vi "Format Address Pads.vi"(4 "WorkTable":refnum<class "WorkTable Class.lvclass">, 6 "Sides":T1[](array[typedef]), 8 "error in":errorcluster, 9 "Slot":i32, 10 "Chuck":i32, 11 "Console Log in":refnum<class "Console Log.lvclass">) -> (0 "error out":errorcluster, 2 "Formatted Address Pads":string[](array[string]), 3 "Console Log out":refnum<class "Console Log.lvclass">)   [LabVIEW 2011, in "Console Log.lvclass"]
uses:
  Console Log.lvclass
  Shared Components/Utils/Type Definitions/3d Line.ctl
  Shared Components/Vec3d Class/Vec3d Class.lvclass
  Shared Components/WorkTable Class/WorkTable Class.lvclass
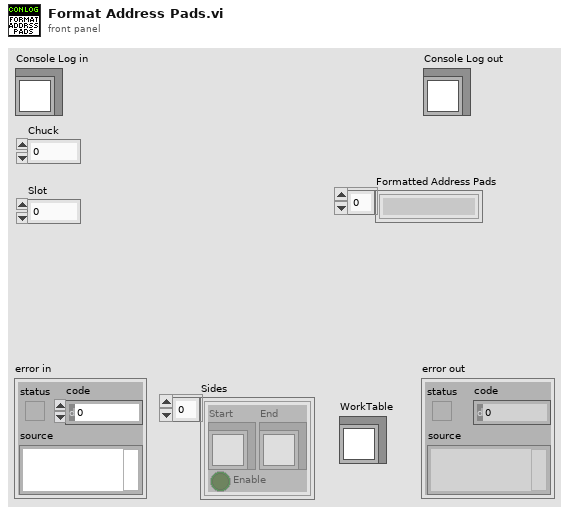
[diagram p1: front panel]
types:
  T1 = typedef "3d Line.ctl" = cluster{"Start":refnum<class "Vec3d Class.lvclass">, "End":refnum<class "Vec3d Class.lvclass">, "Enable":bool}
  T2 = typedef "Worktable_Module Slot.ctl" = cluster{"Slot State":enum16{"Empty", "Bare HDI", "Unglued", "Stamped", "PartOnTop", "Weighted", "Unpotted", "Potted"}, "BBM Type":enum16{"None", "BBM", "GlassSlide"}, "HDI Type":enum16{"None", "HDI", "Polyimide"}, "Vacuum Channel":u8, "Location/Orientation BBM":T3, "Location/Orientation HDI":T3, "S/N":string}
  T3 = typedef "Position_Orientation.ctl" = cluster{"Center":refnum<class "Vec3d Class.lvclass">, "Orientation":refnum<class "Orient3d Class.lvclass">}
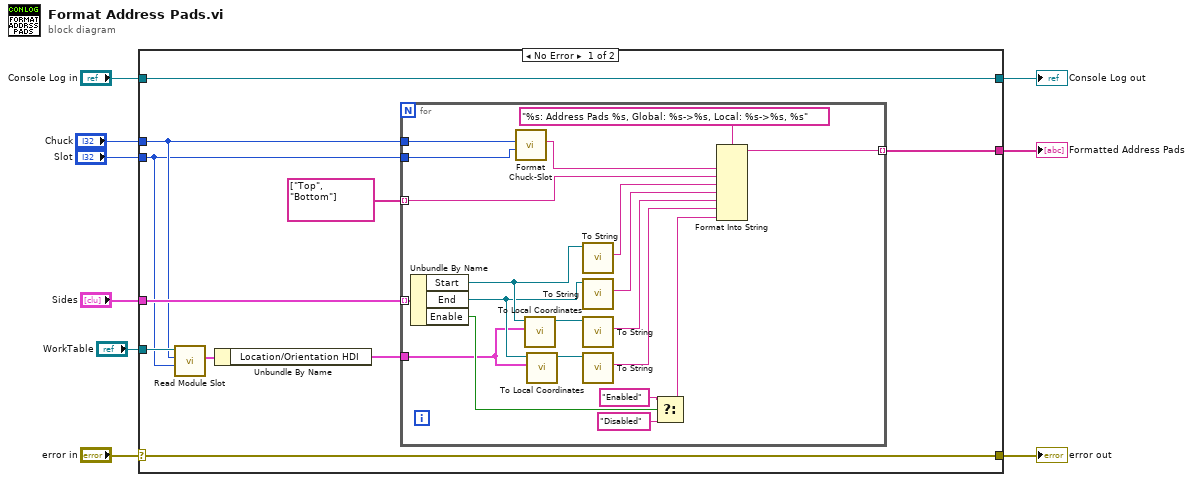
[diagram p0: block diagram]
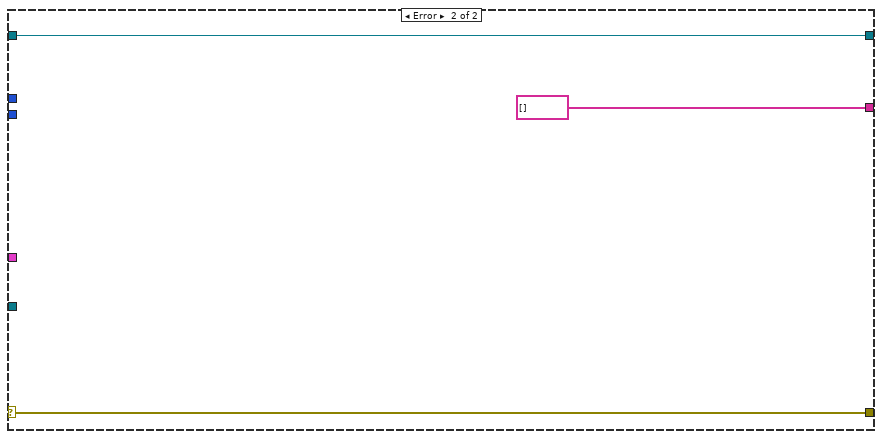
[diagram p2: hidden frame]
diagram:
  n1 = case shown="No Error" "error in" {
    selector: "error in" -> [w18 w42]
    tunnel: [w18 w42] -> w8
    tunnel: [w19 w41] -> w6
    tunnel: "Console Log in" -> [w19 w41]
    tunnel: "Sides" -> [w17 _]
    tunnel: [w16 string[] []] -> w4
    tunnel: "Chuck" -> [w13 _]
    tunnel: "Slot" -> [w12 _]
    tunnel: "WorkTable" -> [w14 _]
    frame No Error {
      n2 = call-dynamic "Read Module Slot.vi"("slot"=w12, "chuck"=w13, "WorkTable in"=w14) -> ("Module Slot"=w11:T2)  [unwired: 6 in, 2 out]
      n3 = Unbundle By Name(w11) -> ("Location/Orientation HDI"=w10:T3)
      n4 = for {
        tunnel: w17 -> [w39] mode=indexing
        tunnel: [w32] -> w16 mode=indexing
        tunnel: string[] ["Top", "Bottom"] -> [w31] mode=indexing
        tunnel: w13 -> [w28]
        tunnel: w12 -> [w27]
        tunnel: w10 -> [w22]
        n5 = Unbundle By Name(w39) -> ("Start"=w24:refnum<class "Vec3d Class.lvclass">, "End"=w23:refnum<class "Vec3d Class.lvclass">, "Enable"=w38:bool)
        n6 = call "Format Chuck-Slot.vi"("Slot"=w27, "Chuck"=w28) -> ("Formatted Chuck/Slot"=w30:string)  [unwired: 7 in, 2 out]
        n7 = call "To Local Coordinates.vi"("Center/Orientation"=w22, "Global Coordinates"=w24) -> ("Local Coordinates"=w26:refnum<class "Vec3d Class.lvclass">)  [unwired: 8 in, 1 out]
        n8 = call "To Local Coordinates.vi"("Center/Orientation"=w22, "Global Coordinates"=w23) -> ("Local Coordinates"=w25:refnum<class "Vec3d Class.lvclass">)  [unwired: 8 in, 1 out]
        n9 = call "To String.vi"("Vec3d in"=w24) -> ("Vec3d String"=w34:string)  [unwired: 8 in, 2 out]
        n10 = call "To String.vi"("Vec3d in"=w23) -> ("Vec3d String"=w33:string)  [unwired: 8 in, 2 out]
        n11 = call "To String.vi"("Vec3d in"=w26) -> ("Vec3d String"=w21:string)  [unwired: 8 in, 2 out]
        n12 = call "To String.vi"("Vec3d in"=w25) -> ("Vec3d String"=w20:string)  [unwired: 8 in, 2 out]
        n13 = Select(t="Enabled", s=w38, f="Disabled") -> (s? t:f=w29:string)
        n14 = Format Into String(format string="%s: Address Pads %s, Global: %s->%s, Local: %s->%s, %s", w30, w31, w34, w33, w21, w20, w29) -> (resulting string=w32:string)  [unwired: 2 in, 1 out]
      }
    }
    frame Error {
    }
  }
  "error out" <- w8
  "Console Log out" <- w6
  "Formatted Address Pads" <- w4
